vi "VCO.vi"(0 "System no.":i32=1 min=1 max=4 step=1, 2 "Axes to command":string[](array[string]), 3 "Vel. control mode":bool[](array[boolean]), 5 "error in":errorcluster) -> (19 "error out":errorcluster)   [LabVIEW 2026]
doc: "Sets velocity-control mode for specified axes.\n\nAnalog: Velocity control mode can only be set for all axes equally. Therefore only first field of Vel.control mode is valid.\n\nE-516, E-517, E-518, E-727, E-754: The VCO command saves the parameters in RAM only. To save the currently valid parameters to flash ROM, where they become the power-on defaults, you must run WPA.vi. Parameter changes not saved with WPA will be lost when the controller is powered off.\n\nE-761: The VCO command saves the parameters in RAM only. To save the currently valid parameters to flash ROM, where they become the power-on defaults, you must run WPA.vi with \"Affected axes\" as an empty array. Parameter changes not saved with WPA will be lost when the PC is powered off or the E-761 is rebooted."
panel:
  # "Sets velocity control mode for specified axes."
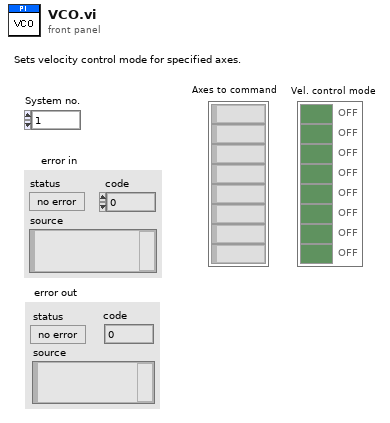
[diagram p1: front panel]
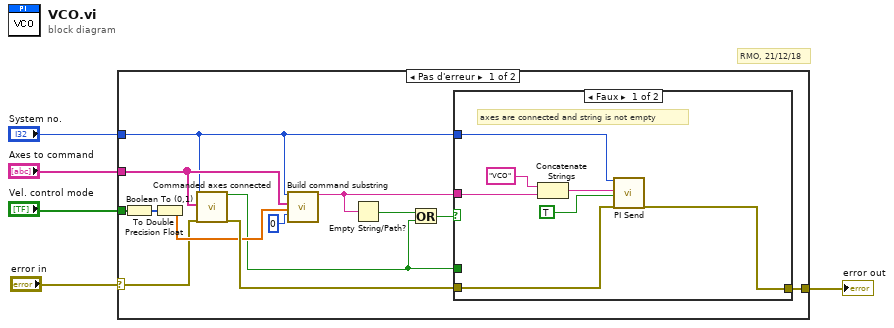
[diagram p0: block diagram]
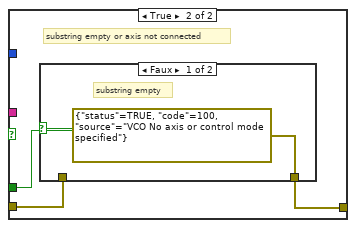
[diagram p2: hidden frame]
diagram:
  # "RMO, 21/12/18"
  n1 = case shown="Pas d'erreur" "error in" {
    selector: "error in" -> [w9 w31]
    tunnel: [w18 w31] -> w5
    tunnel: "System no." -> [w10 _]
    tunnel: "Axes to command" -> [w16 _]
    tunnel: "Vel. control mode" -> [w14 _]
    frame No Error {
      n2 = Boolean To (0,1)(Boolean=w14) -> (0, 1=w13:i16[])
      n3 = To Double Precision Float(number=w13) -> (double precision float=w11:dbl[])
      n4 = call "Commanded axes connected.vi"("System no."=w10, "Commanded axes"=w16, "error in"=w9) -> ("Controller error"=w6:bool, "error out"=w17:errorcluster)  [unwired: 1 in, 14 out]
      n5 = call "Build command substring.vi"("System no."=w10, "Affected axes"=w16, "Parameters"=w11, "No. of digits"=i16 0 ("No.of digits")) -> ("Command substring"=w8:string)  [unwired: 3 in, 12 out]
      n6 = Empty String/Path?(string/path=w8) -> (empty?=w7:bool)
      n7 = Or(x=w7, y=w6) -> (x .or. y?=w15:bool)
      n8 = case shown="Faux" w15 {
        tunnel: w8 -> [w24 _]
        tunnel: [w20 w28] -> w18
        tunnel: w17 -> [w21 w26]
        tunnel: w6 -> [_ w27]
        tunnel: w10 -> [w19 _]
        frame False {
          # "axes are connected and string is not empty"
          n9 = Concatenate Strings("VCO", w24) -> (w22:string)
          n10 = call "PI Send.vi"("System no."=w19, "String to send"=w22, "Attach termination char.?"=TRUE ("Attach Linefeed?"), "error in"=w21) -> ("error out"=w20:errorcluster)  [unwired: 2 in, 13 out]
        }
        frame True {
          # "substring empty or axis not connected"
          n11 = case shown="Faux" w27 {
            tunnel: [errorcluster {"status"=TRUE, "code"=100, "source"="VCO No axis or control mode specified"} ("error out") w30] -> w28
            tunnel: w26 -> [_ w30]
            frame False {
              # "substring empty"
            }
            frame True {
              # "commanded axis not connected"
            }
          }
        }
      }
    }
    frame Error {
    }
  }
  "error out" <- w5
